vi "week5_read-file_LV18.vi"() -> ()   [LabVIEW 2018]
uses:
  <vilib>/Utility/file.llb/Read Delimited Spreadsheet (DBL).vi
  <vilib>/Utility/file.llb/Read Delimited Spreadsheet (string).vi
panel:
  in  "Tab Control":T1(tab)
  in  "Measurement_file_path":path=path "C:/Users/Robert/ownCloud/LabView 101-RI/RI_week4/output_data/meas_file.lvm"
  out "Meas. file last # read from c1":dbl
  out "Meas. file last # read from c2":dbl
  out "Meas. file column 1 Array":ext[](array[numeric]) format="%#_6f"
  in  "CSV_path":path=path "C:/Users/Robert/ownCloud/LabView 101-RI/RI_week4/output_data/write_csv.csv"
  out "CSV file column 1 Array":ext[](array[numeric]) format="%#_6f"
  out "CSV file last # read from c1 2":dbl
  out "CSV file last # read from c1":dbl
  out "CSV all data":dbl[][](array[numeric])
  out "CSV all data 2":dbl[][](array[numeric])
  in  "CSV_text&num_path":path=path "C:/Users/Robert/ownCloud/LabView 101-RI/RI_week5/example_file.csv"
  out "Mixed text & numbers read as DOUBLE":dbl[][](array[numeric])
  out "Mixed text & numbers read as STRING":string[][](array[string])
  out "Mixed text & numbers: numbers only":dbl[][](array[numeric])
  in  "Select example":u16(ring) items=["Read .lvm file", "Read .csv file", "Read mixed string & num"]
  # "<< note, this is an array of \nnumbers"
  # "<< note, this is \nan array of \nstrings"
  # "<< note, this is an array \nof numbers"
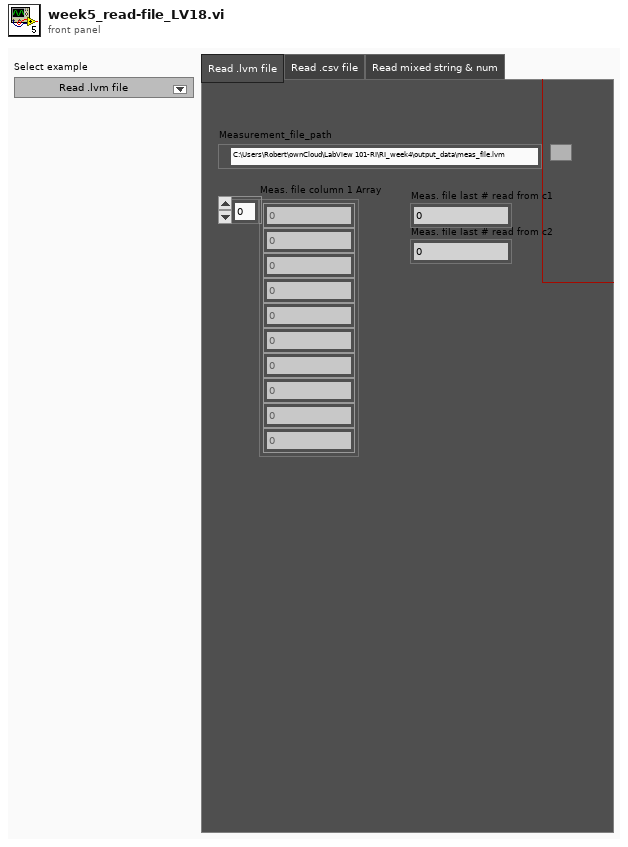
[diagram p1: front panel]
types:
  T1 = enum32{"Read .lvm file", "Read .csv file", "Read mixed string & num"}
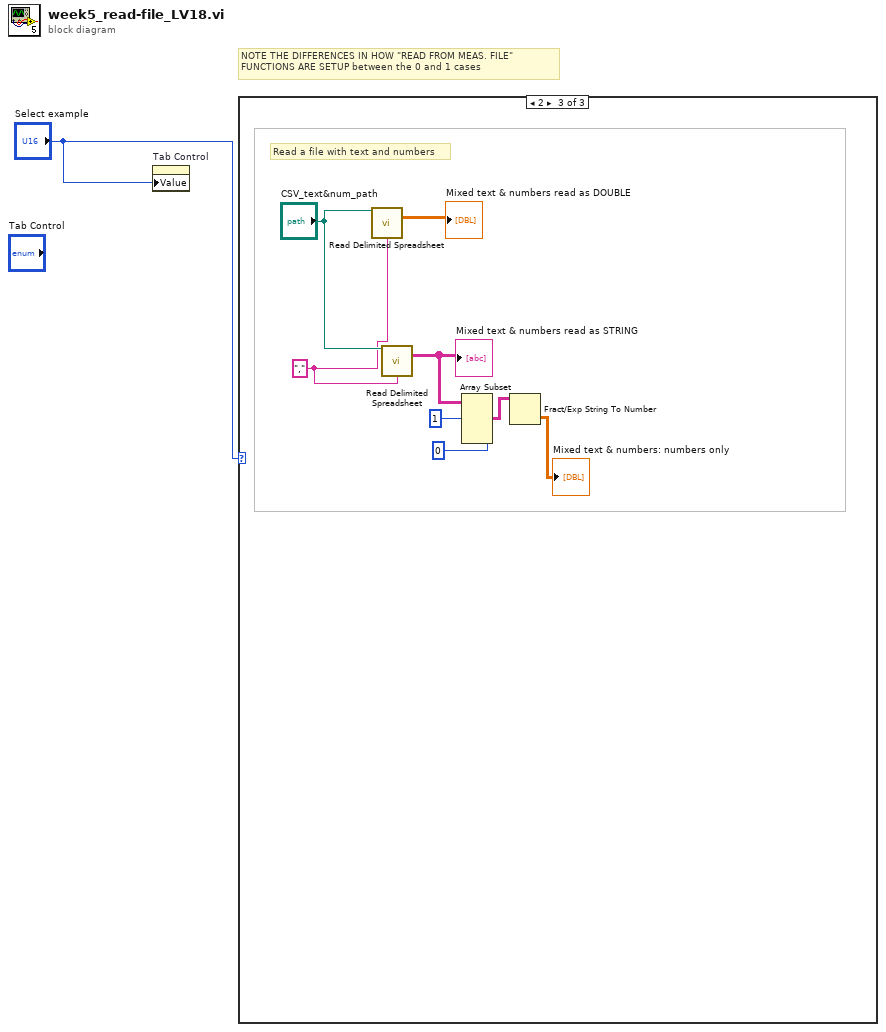
[diagram p0: block diagram]
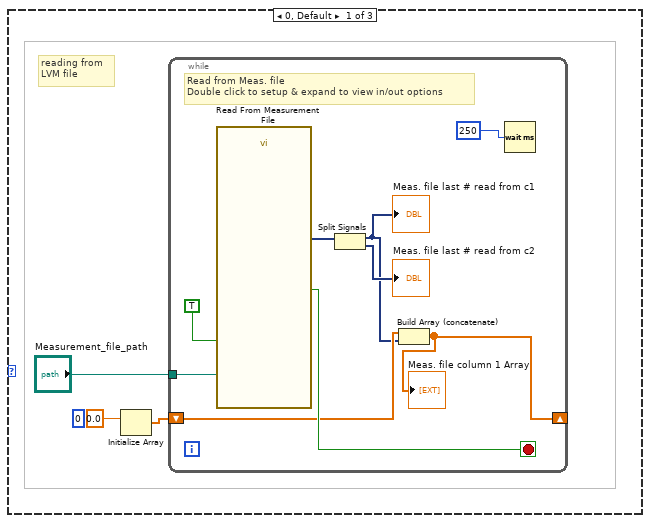
[diagram p2: hidden frame]
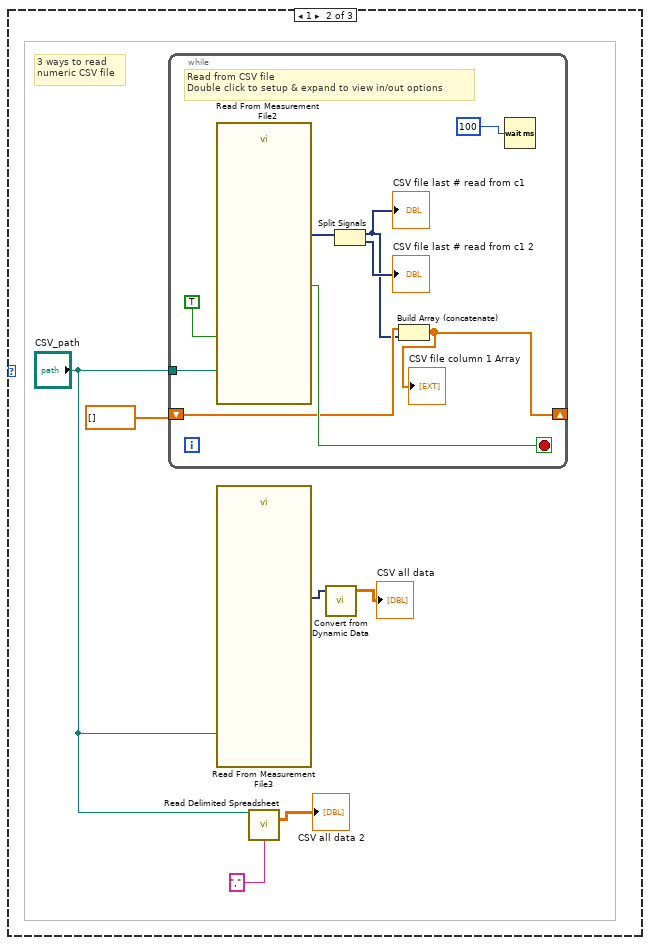
[diagram p3: hidden frame]
diagram:
  # "NOTE THE DIFFERENCES IN HOW \"READ FROM MEAS. FILE\" \nFUNCTIONS ARE SETUP between the 0 and 1 cases"
  n1 = property on="Tab Control" class="TabCtl (strict)"("Value"="Select example") -> ()  [unwired: 2 in, 2 out]
  n2 = case shown="2" "Select example" {
    frame 0, Default {
      (unwired) 0
      # "reading from \nLVM file"
      n3 = Initialize Array(0.0) -> (w4:dbl[])  [unwired: 1 in]
      n4 = while {
        tunnel: "Measurement_file_path" -> [w13]
        shift-right: [w7] -> _
        shift-left: w4 -> [w6]
        stop <- w9 stop-if-true
        # "Read from Meas. file\nDouble click to setup & expand to view in/out options"
        n5 = call "Read From Measurement File"("Filename"=w13, "Enable"=TRUE) -> ("Signals"=w10:dynamicdata, "EOF?"=w9:bool)  [unwired: 4 in, 4 out]
        n6 = Split Signals(w10) -> (w5:dynamicdata, →"Meas. file last # read from c2":dynamicdata)  [unwired: 2 in]
        "Meas. file last # read from c1" <- w5
        n7 = Build Array (concatenate)(w6, w5) -> (w7:dbl[])
        "Meas. file column 1 Array" <- w7
        n8 = Wait (ms)(milliseconds to wait=250) -> ()  [unwired: 1 out]
      }
    }
    frame 1 {
      # "3 ways to read\nnumeric CSV file"
      n9 = while {
        shift-right: [w23] -> _
        shift-left: dbl[] [] -> [w22]
        tunnel: "CSV_path" -> [w20]
        stop <- w25 stop-if-true
        # "Read from CSV file\nDouble click to setup & expand to view in/out options"
        n10 = call "Read From Measurement File2"("Filename"=w20, "Enable"=TRUE) -> ("Signals"=w26:dynamicdata, "EOF?"=w25:bool)  [unwired: 4 in, 4 out]
        n11 = Split Signals(w26) -> (w21:dynamicdata, →"CSV file last # read from c1 2":dynamicdata)  [unwired: 2 in]
        "CSV file last # read from c1" <- w21
        n12 = Build Array (concatenate)(w22, w21) -> (w23:dbl[])
        "CSV file column 1 Array" <- w23
        n13 = Wait (ms)(milliseconds to wait=100) -> ()  [unwired: 1 out]
      }
      n14 = call "Read From Measurement File3"("Filename"="CSV_path") -> ("Signals"=w16:dynamicdata)  [unwired: 5 in, 5 out]
      n15 = call-poly <vilib>:"Read Delimited Spreadsheet.vi"("file path (dialog if empty)"="CSV_path", "delimiter (\\t)"=",") -> ("all rows"=→"CSV all data 2":dbl[][])  [unwired: 8 in, 5 out]
      n16 = call "Convert from Dynamic Data"("Dynamic Data Type"=w16) -> ("Array"=→"CSV all data":dbl[][])  [unwired: 3 in]
    }
    frame 2 {
      w29 = ","
      # "Read a file with text and numbers"
      n17 = call-poly <vilib>:"Read Delimited Spreadsheet.vi"("file path (dialog if empty)"="CSV_text&num_path", "delimiter (\\t)"=w29) -> ("all rows"=→"Mixed text & numbers read as DOUBLE":dbl[][])  [unwired: 8 in, 5 out]
      n18 = call-poly <vilib>:"Read Delimited Spreadsheet.vi"("file path (dialog if empty)"="CSV_text&num_path", "delimiter (\\t)"=w29) -> ("all rows"=w34:string[][])  [unwired: 8 in, 5 out]
      "Mixed text & numbers read as STRING" <- w34
      n19 = Array Subset(array=w34, index (row)=1, index (col)=0) -> (w35:string[][])  [unwired: 2 in]
      n20 = Fract/Exp String To Number(string=w35) -> (number=→"Mixed text & numbers: numbers only":dbl[][])  [unwired: 3 in, 1 out]
    }
  }
